vi "Kroki URL--constant.vi"() -> (1 "Server is UP":bool, 2 "net address":u32, 3 "Kroki Full URL":string)   [LabVIEW 2019, in "SimpleDependencyInspector.lvlib"]
uses:
  SimpleDependencyInspector.lvlib
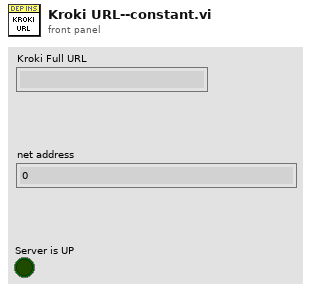
[diagram p1: front panel]
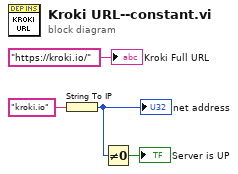
[diagram p0: block diagram]
diagram:
  n1 = String To IP(1:"kroki.io" ("url")) -> (0:w3:u32)
  "net address" <- w3
  n2 = Not Equal To 0?(x=w3) -> (x != 0?=→"Server is UP":bool)
  "Kroki Full URL" <- "https://kroki.io/" ("url")
